vi "Create Pattern Script(Data).vi"(7 "Data Type":T1, 8 "error in (no error)":errorcluster, 10 "Data":u16, 11 "SPI 3W Pattern Creator in":refnum<class "SPI 3W Pattern Creator.lvclass">) -> (0 "error out":errorcluster, 2 "String":string, 3 "SPI 3W Pattern Creator out":refnum<class "SPI 3W Pattern Creator.lvclass">)   [LabVIEW 2018, in "SPI 3W Pattern Creator.lvlib" / "SPI 3W Pattern Creator.lvclass"]
uses:
  SPI 3W Pattern Creator.lvclass
  Protocols/SPI Root Pattern Creator.lvlibp/Plugins/SouceCode/SPI_Pattern Creator/SPI Root/Data Type.ctl
  Interfaces/Protocol Interface.lvlibp/Interfaces/Protocol Interface/Pin State.ctl
  Interfaces/Protocol Interface.lvlibp/Interfaces/Protocol Interface/Protocol Interface.lvclass
  Protocols/SPI Root Pattern Creator.lvlibp/Plugins/SouceCode/SPI_Pattern Creator/SPI Root/SPI Root Pattern Creator.lvclass
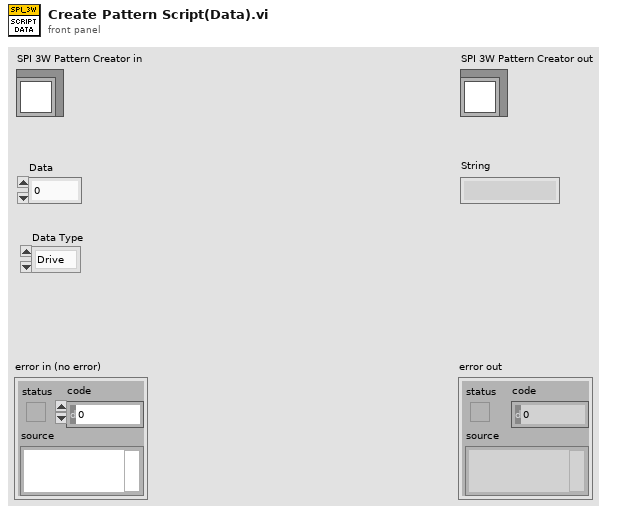
[diagram p1: front panel]
types:
  T1 = typedef "SPI Root Pattern Creator.lvlibp/SPI Root Pattern Creator.lvclass/Data Type.ctl" = enum16{"Drive", "Compare", "Read"}
  T2 = typedef "Protocol Interface.lvlibp/Protocol Interface.lvclass/Pin State.ctl" = enum16{"0", "1", "L", "H", "X", "V", "D", "M"}
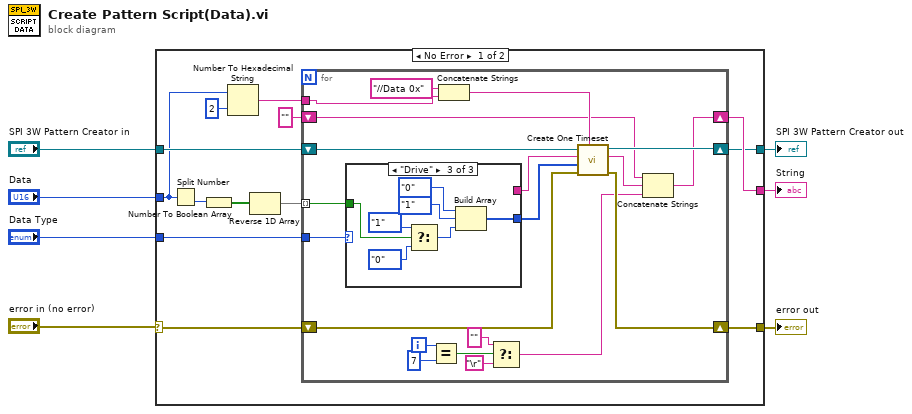
[diagram p0: block diagram]
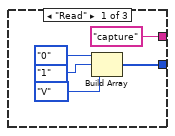
[diagram p2: hidden frame]
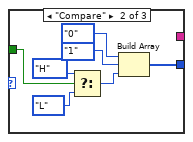
[diagram p3: hidden frame]
diagram:
  n1 = case shown="No Error" "error in (no error)" {
    selector: "error in (no error)" -> [w15 w60]
    tunnel: "Data" -> [w14 _]
    tunnel: "SPI 3W Pattern Creator in" -> [w18 w61]
    tunnel: "Data Type" -> [w16 _]
    tunnel: [w10 _] -> w4
    tunnel: [w9 w61] -> w3
    tunnel: [w8 w60] -> w2
    frame No Error {
      n2 = Split Number(x=w14) -> (lo(x)=w20:u8)  [unwired: 1 out]
      n3 = Number To Boolean Array(number=w20) -> (Boolean array=w19:bool[])
      n4 = Number To Hexadecimal String(1:i16 2 ("width (-)"), 2:w14) -> (0:w12:string)
      n5 = Reverse 1D Array(array=w19) -> (reversed array=w17:bool[])
      n6 = for {
        shift-right: [w31] -> w9
        shift-left: w18 -> [w38]
        tunnel: w17 -> [w39] mode=indexing
        tunnel: w16 -> [w40]
        shift-right: [w27] -> w8
        shift-left: w15 -> [w35]
        tunnel: w12 -> [w33]
        shift-right: [w30] -> w10
        shift-left: "" -> [w29]
        i -> [w26]
        n7 = case shown="\"Drive\"" w40 {
          tunnel: w39 -> [_ w49 w56]
          tunnel: ["capture" _ _] -> w36
          tunnel: [w41 w50 w57] -> w37
          frame "Read" {
            n8 = Build Array(Pin_State."0" ("PinState"), Pin_State."1" ("PinState"), Pin_State."V" ("element")) -> (w41:T2[])
          }
          frame "Compare" {
            n9 = Select(t=Pin_State."H" ("PinState"), s=w49, f=Pin_State."L" ("PinState")) -> (s? t:f=w48:T2)
            n10 = Build Array(Pin_State."0" ("PinState"), Pin_State."1" ("PinState"), w48) -> (w50:T2[])
          }
          frame "Drive" {
            n11 = Select(t=Pin_State."1" ("PinState"), s=w56, f=Pin_State."0" ("PinState")) -> (s? t:f=w55:T2)
            n12 = Build Array(Pin_State."0" ("PinState"), Pin_State."1" ("PinState"), w55) -> (w57:T2[])
          }
        }
        n13 = Equal?(x=w26, y=7) -> (x = y?=w24:bool)
        n14 = Concatenate Strings("//Data 0x" ("string"), w33) -> (w32:string)
        n15 = Select(t="", s=w24, f="\r") -> (s? t:f=w22:string)
        n16 = call-dynamic "Create One Timeset.vi"("Notes"=w32, "error in (no error)"=w35, "PinStates"=w37, "OpCode"=w36, "SPI 3W Pattern Creator in"=w38) -> ("error out"=w27:errorcluster, "String  out"=w28:string, "SPI 3W Pattern Creator out"=w31:refnum<class "SPI 3W Pattern Creator.lvclass">)  [unwired: 4 in]
        n17 = Concatenate Strings(w29, w28, w22) -> (w30:string)
      }
    }
    frame Error {
    }
  }
  "error out" <- w2
  "SPI 3W Pattern Creator out" <- w3
  "String" <- w4
